vi "niFpgaLinearInterpolationTemplate.vi"(0 "y0":fxp<+/-,16,16>, 5 "y1":fxp<+/-,16,16>, 9 "x":fxp<+,16,0> format="%04x") -> (4 "y":fxp<+/-,16,16>)   [LabVIEW 2017]
doc: "Performs linear interpolation to approximate a function evaluation at an arbitrary location in an interval between two known points. The data type you wire to <B>y0</B> determines the output <B>y</B> data type."
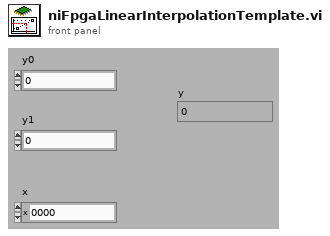
[diagram p1: front panel]
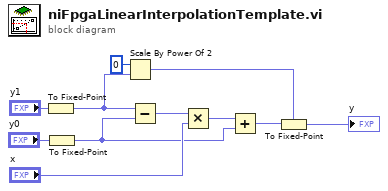
[diagram p0: block diagram]
diagram:
  n1 = To Fixed-Point(number="y1") -> (fixed-point=w4:fxp<+/-,16,16>)  [unwired: 1 in]
  n2 = To Fixed-Point(number="y0") -> (fixed-point=w3:fxp<+/-,16,16>)  [unwired: 1 in]
  n3 = Scale By Power Of 2(n=0, x=w4) -> (x*2^n=w2:fxp<+/-,16,16>)
  n4 = Subtract(x=w4, y=w3) -> (x-y=w11:fxp<+/-,17,17>)
  n5 = Multiply(x=w11, y="x") -> (x*y=w8:fxp<+/-,33,17>)
  n6 = Add(x=w8, y=w3) -> (x+y=w7:fxp<+/-,34,18>)
  n7 = To Fixed-Point(fixed-point type=w2, number=w7) -> (fixed-point=→"y":fxp<+/-,16,16>)
